vi "Control_Tiempo_BIn.vi"(0 "Tiempos ON":T2={"T.M.CH1"=20, "T.M.CH2"=20, "T.M.CH3"=20, "T.M.CH4"=20, "T.M.CH5"=20, "T.M.CH6"=20, "T.M.CH7"=20, "T.M.CH8"=20} {"T.M.CH8" min=1 step=1; "T.M.CH7" min=1 step=1; "T.M.CH6" min=1 step=1; "T.M.CH5" min=1 step=1; "T.M.CH4" min=1 step=1; "T.M.CH3" min=1 step=1; "T.M.CH2" min=1 step=1; "T.M.CH1" min=1 step=1}, 1 "Tiempos OFF":T1={"T.M.CH1"=20, "T.M.CH2"=20, "T.M.CH3"=20, "T.M.CH4"=20, "T.M.CH5"=20, "T.M.CH6"=20, "T.M.CH7"=20, "T.M.CH8"=20} {"T.M.CH8" min=1 step=1; "T.M.CH7" min=1 step=1; "T.M.CH6" min=1 step=1; "T.M.CH5" min=1 step=1; "T.M.CH4" min=1 step=1; "T.M.CH3" min=1 step=1; "T.M.CH2" min=1 step=1; "T.M.CH1" min=1 step=1}, 5 "error in":errorcluster) -> (14 "Estados_Salidas":bool[](array[boolean]), 19 "Error Out":errorcluster)   [LabVIEW 2013]
uses:
  Controles/Tiempos_ON_TB.ctl
  Controles/Tiempos_OFF_TB.ctl
panel:
  # "T. OFF (s)"
  # "T. ON (s)"
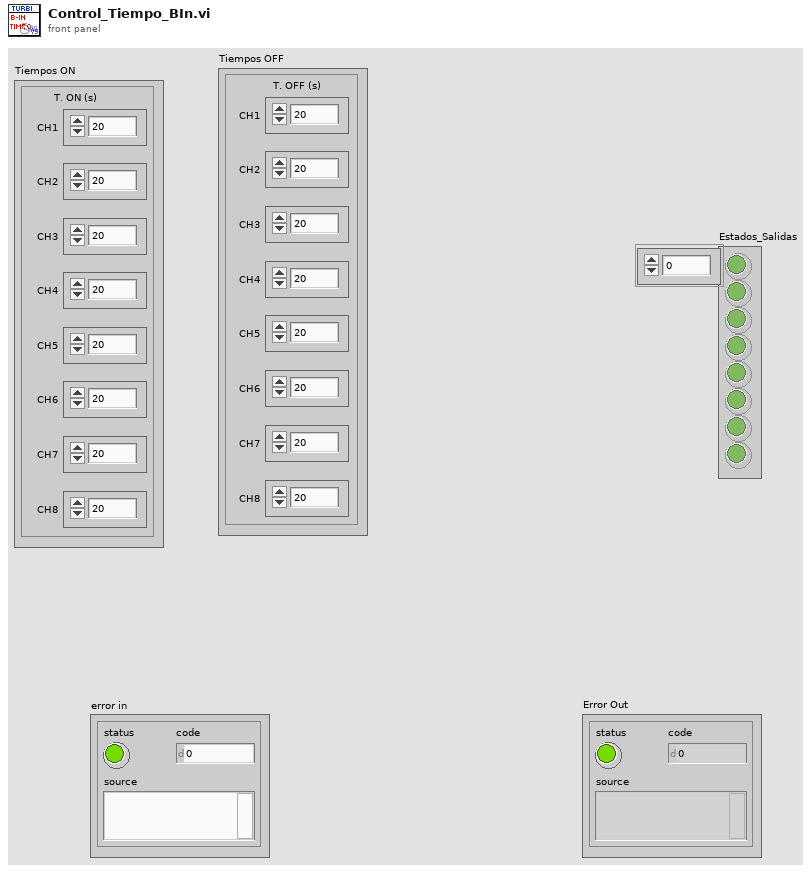
[diagram p1: front panel]
types:
  T1 = typedef "Tiempos_OFF_TB.ctl" = cluster{"T.M.CH1":u16, "T.M.CH2":u16, "T.M.CH3":u16, "T.M.CH4":u16, "T.M.CH5":u16, "T.M.CH6":u16, "T.M.CH7":u16, "T.M.CH8":u16}
  T2 = typedef "Tiempos_ON_TB.ctl" = cluster{"T.M.CH1":u16, "T.M.CH2":u16, "T.M.CH3":u16, "T.M.CH4":u16, "T.M.CH5":u16, "T.M.CH6":u16, "T.M.CH7":u16, "T.M.CH8":u16}
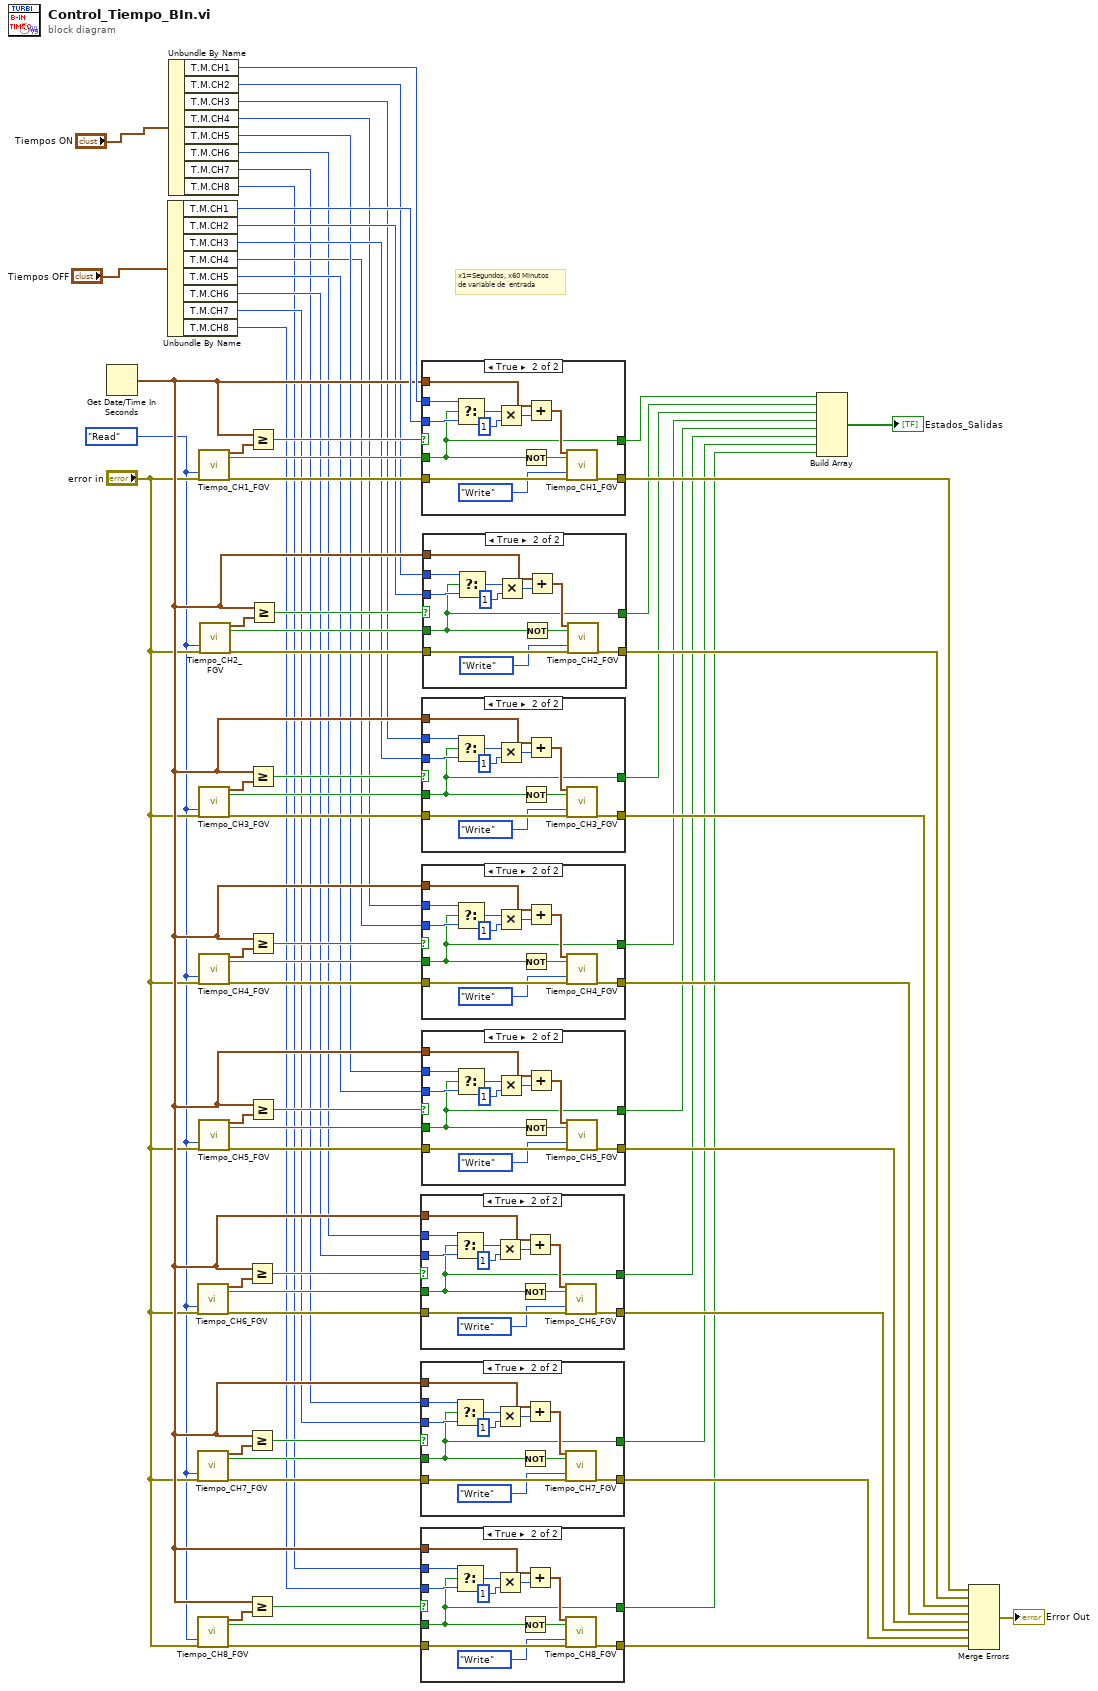
[diagram p0: block diagram]
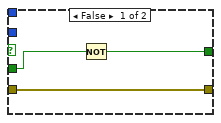
[diagram p2: hidden frame]
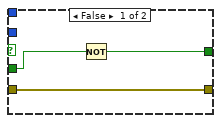
[diagram p3: hidden frame]
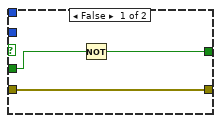
[diagram p4: hidden frame]
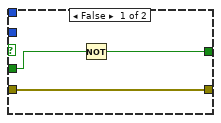
[diagram p5: hidden frame]
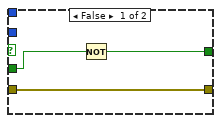
[diagram p6: hidden frame]
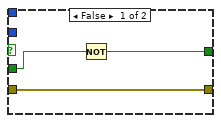
[diagram p7: hidden frame]
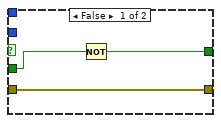
[diagram p8: hidden frame]
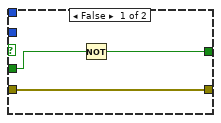
[diagram p9: hidden frame]
diagram:
  w21 = enum16{"Write", "Read"}."Read" ("Opción")
  # "x1=Segundos, x60 Minutos\nde variable de  entrada"
  n1 = Get Date/Time In Seconds() -> (seconds since 1Jan1904=w37:timestamp)
  n2 = Unbundle By Name("Tiempos OFF") -> ("T.M.CH1"=w67:u16, "T.M.CH2"=w35:u16, "T.M.CH3"=w33:u16, "T.M.CH4"=w30:u16, "T.M.CH5"=w29:u16, "T.M.CH6"=w27:u16, "T.M.CH7"=w25:u16, "T.M.CH8"=w23:u16)
  n3 = Unbundle By Name("Tiempos ON") -> ("T.M.CH1"=w68:u16, "T.M.CH2"=w36:u16, "T.M.CH3"=w34:u16, "T.M.CH4"=w32:u16, "T.M.CH5"=w31:u16, "T.M.CH6"=w28:u16, "T.M.CH7"=w26:u16, "T.M.CH8"=w24:u16)
  n4 = call "Tiempo_CH6_FGV.vi"("Opción"=w21, "Error In"="error in") -> ("Tiempo_OUT"=w38:timestamp, "Prox. Estado_OUT"=w40:bool, "Error Out"=w41:errorcluster)  [unwired: 15 in]
  n5 = call "Tiempo_CH7_FGV.vi"("Opción"=w21, "Error In"="error in") -> ("Tiempo_OUT"=w45:timestamp, "Prox. Estado_OUT"=w43:bool, "Error Out"=w42:errorcluster)  [unwired: 15 in]
  n6 = call "Tiempo_CH8_FGV.vi"("Opción"=w21, "Error In"="error in") -> ("Tiempo_OUT"=w46:timestamp, "Prox. Estado_OUT"=w48:bool, "Error Out"=w49:errorcluster)  [unwired: 15 in]
  n7 = call "Tiempo_CH1_FGV.vi"("Opción"=w21, "Error In"="error in") -> ("Tiempo_OUT"=w71:timestamp, "Prox. Estado_OUT"=w69:bool, "Error Out"=w66:errorcluster)  [unwired: 15 in]
  n8 = call "Tiempo_CH3_FGV.vi"("Opción"=w21, "Error In"="error in") -> ("Tiempo_OUT"=w61:timestamp, "Prox. Estado_OUT"=w59:bool, "Error Out"=w58:errorcluster)  [unwired: 15 in]
  n9 = call "Tiempo_CH4_FGV.vi"("Opción"=w21, "Error In"="error in") -> ("Tiempo_OUT"=w54:timestamp, "Prox. Estado_OUT"=w56:bool, "Error Out"=w57:errorcluster)  [unwired: 15 in]
  n10 = call "Tiempo_CH5_FGV.vi"("Opción"=w21, "Error In"="error in") -> ("Tiempo_OUT"=w53:timestamp, "Prox. Estado_OUT"=w51:bool, "Error Out"=w50:errorcluster)  [unwired: 15 in]
  n11 = call "Tiempo_CH2_FGV.vi"("Opción"=w21, "Error In"="error in") -> ("Tiempo_OUT"=w62:timestamp, "Prox. Estado_OUT"=w64:bool, "Error Out"=w65:errorcluster)  [unwired: 15 in]
  n12 = Greater Or Equal?(x=w37, y=w38) -> (x >= y?=w39:bool)
  n13 = Greater Or Equal?(x=w37, y=w45) -> (x >= y?=w44:bool)
  n14 = Greater Or Equal?(x=w37, y=w46) -> (x >= y?=w47:bool)
  n15 = Greater Or Equal?(x=w37, y=w71) -> (x >= y?=w70:bool)
  n16 = Greater Or Equal?(x=w37, y=w61) -> (x >= y?=w60:bool)
  n17 = Greater Or Equal?(x=w37, y=w54) -> (x >= y?=w55:bool)
  n18 = Greater Or Equal?(x=w37, y=w53) -> (x >= y?=w52:bool)
  n19 = Greater Or Equal?(x=w37, y=w62) -> (x >= y?=w63:bool)
  n20 = case shown="True" w39 {
    tunnel: w40 -> [w74 w76]
    tunnel: w28 -> [_ w86]
    tunnel: w27 -> [_ w85]
    tunnel: w41 -> [w72 w84]
    tunnel: [w72 w78] -> w15
    tunnel: [w73 w76] -> w5
    tunnel: w37 -> [_ w75]
    frame False {
      n21 = Not(x=w74) -> (.not. x?=w73:bool)
    }
    frame True {
      n22 = Select(t=w86, s=w76, f=w85) -> (s? t:f=w77:u16)
      n23 = Multiply(x=w77, y=u16 1) -> (x*y=w82:u16)
      n24 = Not(x=w76) -> (.not. x?=w79:bool)
      n25 = Add(x=w75, y=w82) -> (x+y=w81:timestamp)
      n26 = call "Tiempo_CH6_FGV.vi"("Tiempo_IN"=w81, "Prox. Estado_IN"=w79, "Opción"=enum16{"Write", "Read"}."Write", "Error In"=w84) -> ("Error Out"=w78:errorcluster)  [unwired: 13 in, 2 out]
    }
  }
  n27 = case shown="True" w44 {
    tunnel: w43 -> [w89 w91]
    tunnel: w26 -> [_ w101]
    tunnel: w25 -> [_ w100]
    tunnel: w42 -> [w87 w99]
    tunnel: [w87 w93] -> w14
    tunnel: [w88 w91] -> w4
    tunnel: w37 -> [_ w90]
    frame False {
      n28 = Not(x=w89) -> (.not. x?=w88:bool)
    }
    frame True {
      n29 = Select(t=w101, s=w91, f=w100) -> (s? t:f=w92:u16)
      n30 = Multiply(x=w92, y=u16 1) -> (x*y=w97:u16)
      n31 = Not(x=w91) -> (.not. x?=w94:bool)
      n32 = Add(x=w90, y=w97) -> (x+y=w96:timestamp)
      n33 = call "Tiempo_CH7_FGV.vi"("Tiempo_IN"=w96, "Prox. Estado_IN"=w94, "Opción"=enum16{"Write", "Read"}."Write", "Error In"=w99) -> ("Error Out"=w93:errorcluster)  [unwired: 13 in, 2 out]
    }
  }
  n34 = case shown="True" w47 {
    tunnel: w48 -> [w104 w106]
    tunnel: w24 -> [_ w116]
    tunnel: w23 -> [_ w115]
    tunnel: w49 -> [w102 w114]
    tunnel: [w102 w108] -> w13
    tunnel: [w103 w106] -> w3
    tunnel: w37 -> [_ w105]
    frame False {
      n35 = Not(x=w104) -> (.not. x?=w103:bool)
    }
    frame True {
      n36 = Select(t=w116, s=w106, f=w115) -> (s? t:f=w107:u16)
      n37 = Multiply(x=w107, y=u16 1) -> (x*y=w112:u16)
      n38 = Not(x=w106) -> (.not. x?=w109:bool)
      n39 = Add(x=w105, y=w112) -> (x+y=w111:timestamp)
      n40 = call "Tiempo_CH8_FGV.vi"("Tiempo_IN"=w111, "Prox. Estado_IN"=w109, "Opción"=enum16{"Write", "Read"}."Write", "Error In"=w114) -> ("Error Out"=w108:errorcluster)  [unwired: 13 in, 2 out]
    }
  }
  n41 = case shown="True" w70 {
    tunnel: w69 -> [w119 w121]
    tunnel: w68 -> [_ w131]
    tunnel: w67 -> [_ w130]
    tunnel: w66 -> [w117 w129]
    tunnel: [w117 w123] -> w20
    tunnel: [w118 w121] -> w10
    tunnel: w37 -> [_ w120]
    frame False {
      n42 = Not(x=w119) -> (.not. x?=w118:bool)
    }
    frame True {
      n43 = Select(t=w131, s=w121, f=w130) -> (s? t:f=w122:u16)
      n44 = Multiply(x=w122, y=u16 1) -> (x*y=w127:u16)
      n45 = Not(x=w121) -> (.not. x?=w124:bool)
      n46 = Add(x=w120, y=w127) -> (x+y=w126:timestamp)
      n47 = call "Tiempo_CH1_FGV.vi"("Tiempo_IN"=w126, "Prox. Estado_IN"=w124, "Opción"=enum16{"Write", "Read"}."Write", "Error In"=w129) -> ("Error Out"=w123:errorcluster)  [unwired: 13 in, 2 out]
    }
  }
  n48 = case shown="True" w60 {
    tunnel: w59 -> [w134 w136]
    tunnel: w34 -> [_ w146]
    tunnel: w33 -> [_ w145]
    tunnel: w58 -> [w132 w144]
    tunnel: [w132 w138] -> w18
    tunnel: [w133 w136] -> w8
    tunnel: w37 -> [_ w135]
    frame False {
      n49 = Not(x=w134) -> (.not. x?=w133:bool)
    }
    frame True {
      n50 = Select(t=w146, s=w136, f=w145) -> (s? t:f=w137:u16)
      n51 = Multiply(x=w137, y=u16 1) -> (x*y=w142:u16)
      n52 = Not(x=w136) -> (.not. x?=w139:bool)
      n53 = Add(x=w135, y=w142) -> (x+y=w141:timestamp)
      n54 = call "Tiempo_CH3_FGV.vi"("Tiempo_IN"=w141, "Prox. Estado_IN"=w139, "Opción"=enum16{"Write", "Read"}."Write", "Error In"=w144) -> ("Error Out"=w138:errorcluster)  [unwired: 13 in, 2 out]
    }
  }
  n55 = case shown="True" w55 {
    tunnel: w56 -> [w149 w151]
    tunnel: w32 -> [_ w161]
    tunnel: w30 -> [_ w160]
    tunnel: w57 -> [w147 w159]
    tunnel: [w147 w153] -> w17
    tunnel: [w148 w151] -> w7
    tunnel: w37 -> [_ w150]
    frame False {
      n56 = Not(x=w149) -> (.not. x?=w148:bool)
    }
    frame True {
      n57 = Select(t=w161, s=w151, f=w160) -> (s? t:f=w152:u16)
      n58 = Multiply(x=w152, y=u16 1) -> (x*y=w157:u16)
      n59 = Not(x=w151) -> (.not. x?=w154:bool)
      n60 = Add(x=w150, y=w157) -> (x+y=w156:timestamp)
      n61 = call "Tiempo_CH4_FGV.vi"("Tiempo_IN"=w156, "Prox. Estado_IN"=w154, "Opción"=enum16{"Write", "Read"}."Write", "Error In"=w159) -> ("Error Out"=w153:errorcluster)  [unwired: 13 in, 2 out]
    }
  }
  n62 = case shown="True" w52 {
    tunnel: w51 -> [w164 w166]
    tunnel: w31 -> [_ w176]
    tunnel: w29 -> [_ w175]
    tunnel: w50 -> [w162 w174]
    tunnel: [w162 w168] -> w16
    tunnel: [w163 w166] -> w6
    tunnel: w37 -> [_ w165]
    frame False {
      n63 = Not(x=w164) -> (.not. x?=w163:bool)
    }
    frame True {
      n64 = Select(t=w176, s=w166, f=w175) -> (s? t:f=w167:u16)
      n65 = Multiply(x=w167, y=u16 1) -> (x*y=w172:u16)
      n66 = Not(x=w166) -> (.not. x?=w169:bool)
      n67 = Add(x=w165, y=w172) -> (x+y=w171:timestamp)
      n68 = call "Tiempo_CH5_FGV.vi"("Tiempo_IN"=w171, "Prox. Estado_IN"=w169, "Opción"=enum16{"Write", "Read"}."Write", "Error In"=w174) -> ("Error Out"=w168:errorcluster)  [unwired: 13 in, 2 out]
    }
  }
  n69 = case shown="True" w63 {
    tunnel: w64 -> [w179 w181]
    tunnel: w36 -> [_ w191]
    tunnel: w35 -> [_ w190]
    tunnel: w65 -> [w177 w189]
    tunnel: [w177 w183] -> w19
    tunnel: [w178 w181] -> w9
    tunnel: w37 -> [_ w180]
    frame False {
      n70 = Not(x=w179) -> (.not. x?=w178:bool)
    }
    frame True {
      n71 = Select(t=w191, s=w181, f=w190) -> (s? t:f=w182:u16)
      n72 = Multiply(x=w182, y=u16 1) -> (x*y=w187:u16)
      n73 = Not(x=w181) -> (.not. x?=w184:bool)
      n74 = Add(x=w180, y=w187) -> (x+y=w186:timestamp)
      n75 = call "Tiempo_CH2_FGV.vi"("Tiempo_IN"=w186, "Prox. Estado_IN"=w184, "Opción"=enum16{"Write", "Read"}."Write", "Error In"=w189) -> ("Error Out"=w183:errorcluster)  [unwired: 13 in, 2 out]
    }
  }
  n76 = Build Array(w10, w9, w8, w7, w6, w5, w4, w3) -> (→"Estados_Salidas":bool[])
  n77 = Merge Errors(w20, w19, w18, w17, w16, w15, w14, w13) -> (→"Error Out":errorcluster)
